vi "Find Object Item (single) by Path.vi"(7 "Item Path":string, 8 "error in (no error)":errorcluster, 10 "Starting Offset":i32, 11 "JSON":string) -> (0 "error out":errorcluster, 1 "<JSON>":string caption="JSON substring", 2 "Item offset":i32, 3 "Found":bool)   [LabVIEW 2015, in "JSONtext.lvlib"]
uses:
  JSONtext.lvlib
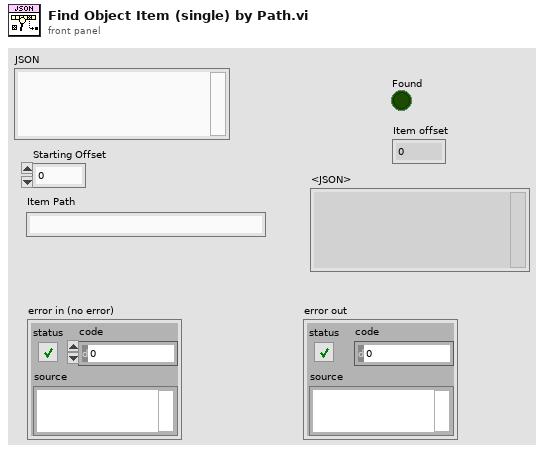
[diagram p1: front panel]
types:
  T1 = typedef "JSONtext.lvlib/Found Items.ctl" = cluster{"Item offset":i32, "Offset past Item":i32, "Name offset":i32, "Offset past Name":i32, "Found":bool, "Empty Object":bool}
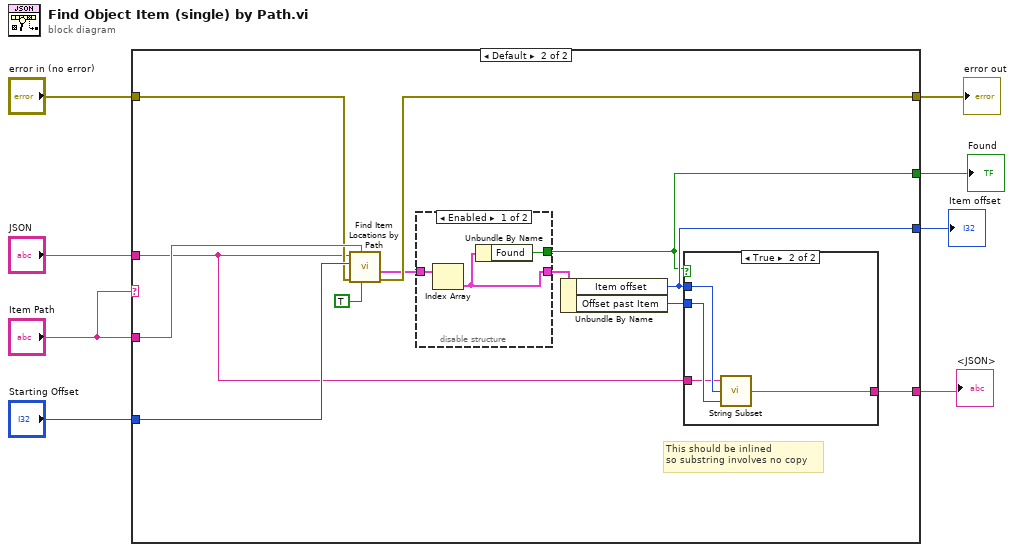
[diagram p0: block diagram]
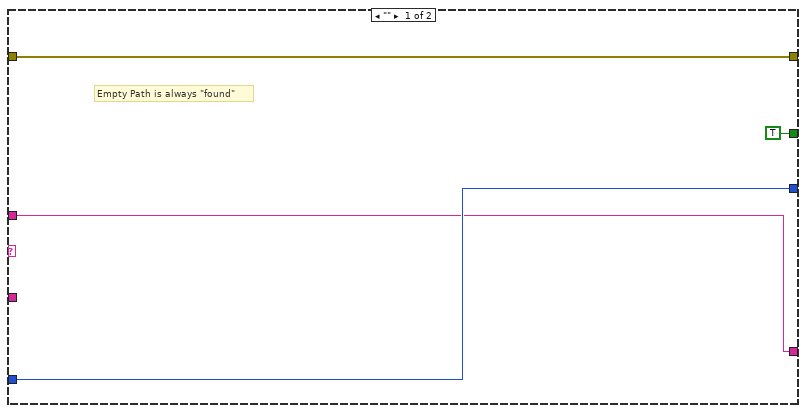
[diagram p2: hidden frame]
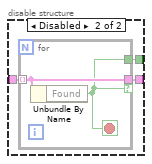
[diagram p3: hidden frame]
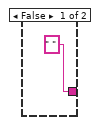
[diagram p4: hidden frame]
diagram:
  n1 = case shown="Default" "Item Path" {
    tunnel: "Item Path" -> [_ w24]
    tunnel: "Starting Offset" -> [w11 w23]
    tunnel: "error in (no error)" -> [w12 w22]
    tunnel: [w12 w21] -> w6
    tunnel: "JSON" -> [w9 w20]
    tunnel: [w11 w16] -> w4
    tunnel: [TRUE ("Found") w13] -> w3
    tunnel: [w9 w14] -> w2
    frame "" {
      # "Empty Path is always \"found\""
    }
    frame Default {
      # "This should be inlined\nso substring involves no copy"
      n2 = call "Find Item Locations by Path.vi"("Only return first found"=TRUE, "Path"=w24, "error in (no error)"=w22, "Object Offset"=w23, "JSON"=w20) -> ("error out"=w21:errorcluster, "Items"=w18:T1[])  [unwired: 5 in]
      n3 = disable-structure shown="Enabled" {
        disable-tunnel: w18 -> [w27 w30]
        disable-tunnel: [w26 w29] -> w17
        disable-tunnel: [w25 w28] -> w13
        frame Enabled {
          n4 = Index Array(array=w27) -> (element=w26:T1)  [unwired: 1 in]
          n5 = Unbundle By Name(w26) -> ("Found"=w25:bool)
        }
        frame Disabled {
          n6 = for {
            tunnel: w30 -> [w32] mode=indexing
            tunnel: [w32] -> w29 if=w31
            tunnel: [w31] -> w28
            stop <- w31 stop-if-true
            n7 = Unbundle By Name(w32) -> ("Found"=w31:bool)
          }
        }
      }
      n8 = Unbundle By Name(w17) -> ("Item offset"=w16:i32, "Offset past Item"=w15:i32)
      n9 = case shown="True" w13 {
        tunnel: w20 -> [_ w34]
        tunnel: [" " ("substring") w37] -> w14
        tunnel: w16 -> [_ w36]
        tunnel: w15 -> [_ w35]
        frame False {
        }
        frame True {
          n10 = call "String Subset.vi"("Offset past End"=w35, "Start offset"=w36, "JSON"=w34) -> ("substring"=w37:string)  [unwired: 2 in]
        }
      }
    }
  }
  "error out" <- w6
  "<JSON>" <- w2
  "Found" <- w3
  "Item offset" <- w4
